vi "Initialise.vi"(8 "error in (no error)":errorcluster, 11 "Renderer":u32) -> (0 "error out":errorcluster, 3 "Asteroid out":refnum<class "Asteroid.lvclass">)   [LabVIEW 2021, in "Asteroid.lvclass"]
uses:
  Asteroid.lvclass
  C:/dev/LabVIEW/LabMelee/Source/Application Specific/Element/Element.lvclass
  Asteroid.lvclass/Asteroid.ctl
  <vilib>/numeric/Random Number (Range) DBL.vi
  <vilib>/Utility/file.llb/Application Directory.vi
  <userlib>/_OpenG.lib/numeric/numeric.llb/Random Number Within Range - I32__ogtk.vi
  <userlib>/_OpenG.lib/numeric/numeric.llb/Random Number Within Range - DBL__ogtk.vi
  Re-use Libraries/Vector 2D/Vector 2D.lvclass
  <userlib>/_OpenG.lib/numeric/numeric.llb/openg_numeric__ogtk.lvlib
  Element/Element.lvclass
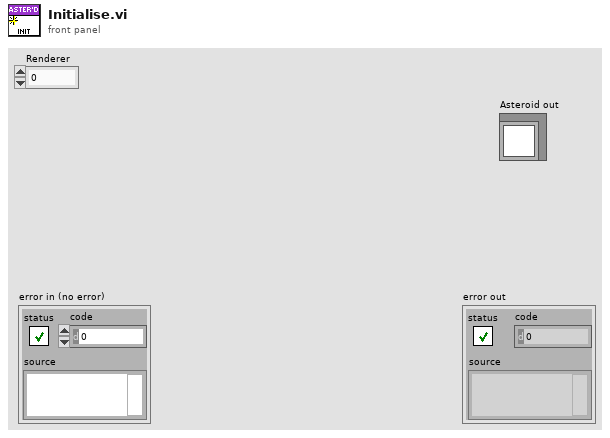
[diagram p1: front panel]
types:
  T1 = typedef "Constants.ctl" = cluster{"Colours":cluster{"OK":u32, "Warning":u32, "Error":u32, "Red":u32, "Green":u32, "Blue":u32, "Yellow":u32}, "System":cluster{"Target Frames Second":dbl, "Windows Size":refnum<class "Vector 2D.lvclass">, "World Size":refnum<class "Vector 2D.lvclass">, "Battle Area Size":refnum<class "Vector 2D.lvclass">, "Sidebar Width":sgl, "SC2 Frame Rate [Seconds/Frame]":sgl, "Sidebar Player 2 Y Offset":sgl}, "Game":cluster{"Maximum Asteroids":i32, "Max Energy":i32, "Max Crew":i32, "Maximum Stars":i32}}
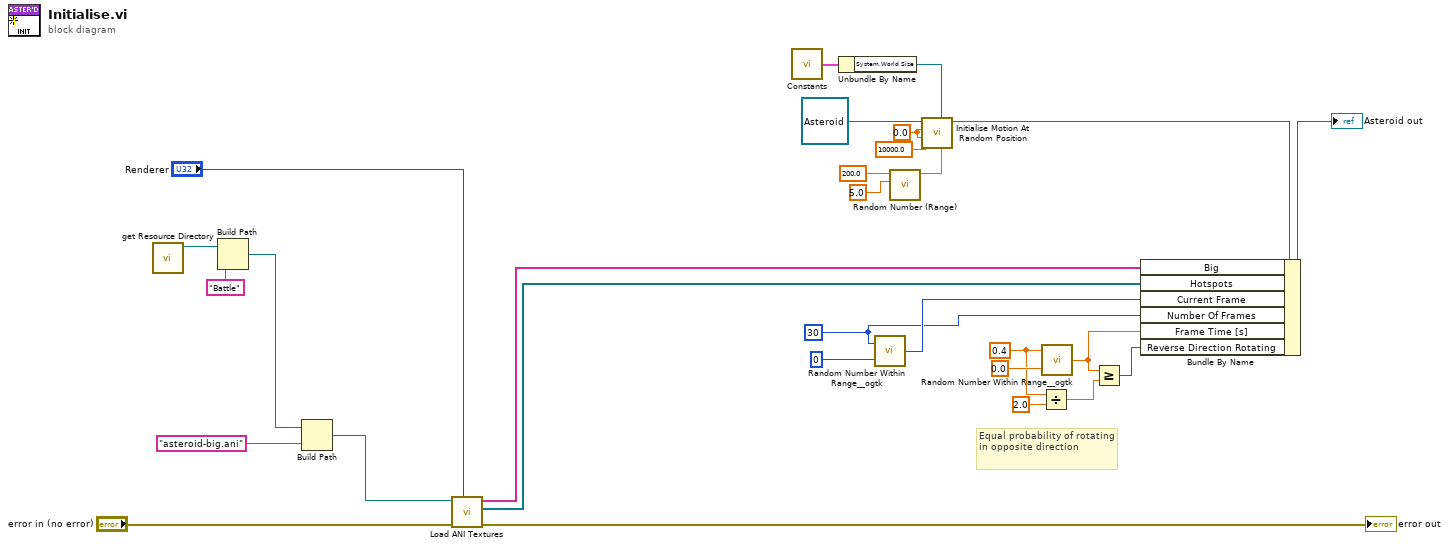
[diagram p0: block diagram]
diagram:
  w5 = sgl 0.0 ("Turn Rate [deg/s]")
  w13 = 0.4 ("High")
  w17 = 30 ("Number Of Frames")
  # "Equal probability of rotating in opposite direction"
  n1 = call "get Resource Directory.vi"() -> ("Resource Directory"=w23:path)  [unwired: 11 in]
  n2 = Build Path(base path=w23, name or relative path="Battle") -> (appended path=w22:path)
  n3 = Build Path(base path=w22, name or relative path="asteroid-big.ani" ("format string")) -> (appended path=w16:path)
  n4 = call "Load ANI Textures.vi"("Renderer"="Renderer", "error in (no error)"="error in (no error)", "Path"=w16) -> ("error out"=→"error out":errorcluster, "Hotspots"=w8:refnum<class "Vector 2D.lvclass">[], "Names"=w9:string[])  [unwired: 6 in]
  n5 = call "Constants.vi"() -> ("Constants"=w21:T1)
  n6 = Unbundle By Name(w21) -> ("System.World Size"=w20:refnum<class "Vector 2D.lvclass">)
  n7 = call-poly <userlib>:"Random Number Within Range__ogtk.vi"("High"=w17, "Low"=0 ("Number Of Frames")) -> ("Random Number"=w18:i32)  [unwired: 3 in]
  n8 = call-poly <vilib>:"Random Number (Range).vi"("lower bound (0)"=sgl 5.0 ("Initial Heading [deg]"), "upper bound (100)"=sgl 200.0 ("Initial Heading [deg]")) -> ("number"=w1:dbl)  [unwired: 9 in]
  n9 = call "Initialise Motion At Random Position.vi"("Initial Velocity [m/s]"=w1, "Field Size"=w20, "Maximum Velocity [m/s]"=sgl 10000.0, "Acceleration [m/s/s]"=w5, "Turn Rate [deg/s]"=w5, "Element in"=refnum<class "Asteroid.lvclass"> refnum ("Asteroid in")) -> ("Element out"=w26:refnum<class "Asteroid.lvclass">)  [unwired: 5 in]
  n10 = Divide(x=w13, y=2.0) -> (x/y=w11:dbl)
  n11 = call-poly <userlib>:"Random Number Within Range__ogtk.vi"("High"=w13, "Low"=0.0) -> ("Random Number"=w14:dbl)  [unwired: 3 in]
  n12 = Greater Or Equal?(x=w14, y=w11) -> (x >= y?=w10:bool)
  n13 = Bundle By Name(cluster=w26, "Big"=w9, "Hotspots"=w8, "Current Frame"=w18, "Number Of Frames"=w17, "Frame Time [s]"=w14, "Reverse Direction Rotating"=w10) -> (→"Asteroid out":refnum<class "Asteroid.lvclass">)
